vi "Do.vi"(8 "error in (no error)":errorcluster, 10 "Actor in":refnum<class "Actor.lvclass">, 11 "Initialize Msg":refnum<class "Initialize Work Msg.lvclass">) -> (0 "error out":errorcluster, 2 "Actor out":refnum<class "Actor.lvclass">)   [LabVIEW 2021, in "Initialize Work Msg.lvclass"]
doc: "This VI delivers the message to the actor by calling the appropriate method(s) on the actor."
uses:
  Initialize Work Msg.lvclass
  Initialize Work Msg.lvclass/Initialize Work Msg.ctl
  Woker Interface/Worker.lvclass
  38615d65-fe0a-408a-ba5f-f88dbd155317.vi
  <vilib>/ActorFramework/Actor/Actor.lvclass
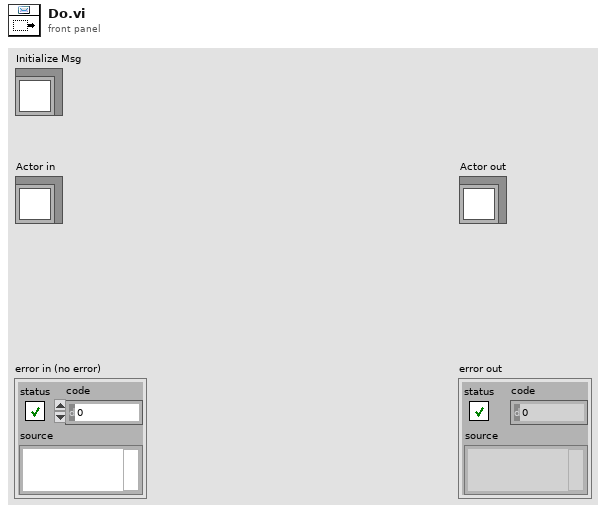
[diagram p1: front panel]
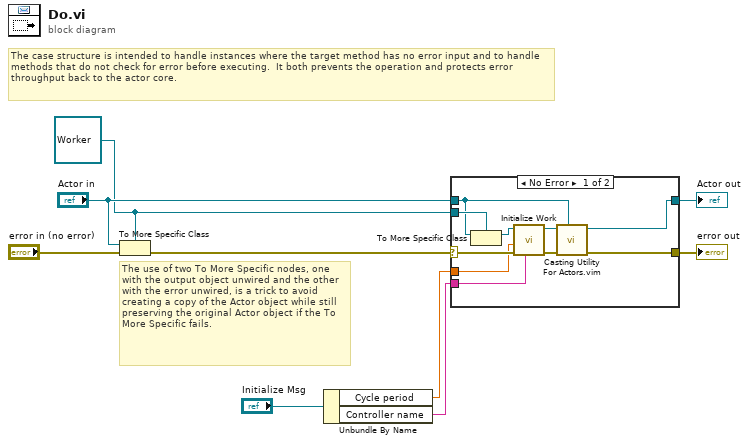
[diagram p0: block diagram]
diagram:
  w4 = refnum<class "Worker.lvclass"> refnum ("Actor in")
  # "The use of two To More Specific nodes, one with the output object unwired and the other with the error unwired, is a trick to avoid creating a copy of the Actor object while still preserving the original Actor object if the To More Specific fails."
  # "The case structure is intended to handle instances where the target method has no error input and to handle methods that do not check for error before executing.  It both prevents the operation and protects error throughput back to the actor core."
  n1 = To More Specific Class(target class=w4, reference="Actor in", error in="error in (no error)") -> (error out=w8:errorcluster)  [unwired: 1 out]
  n2 = Unbundle By Name("Initialize Msg") -> ("Cycle period"=w2:dbl, "Controller name"=w1:string)
  n3 = case shown="No Error" w8 {
    selector: w8 -> [w19 w21]
    tunnel: [w13 w21] -> w7
    tunnel: [w11 w20] -> w6
    tunnel: "Actor in" -> [w10 w20]
    tunnel: w4 -> [w18 _]
    tunnel: w2 -> [w16 _]
    tunnel: w1 -> [w15 _]
    frame No Error {
      n4 = To More Specific Class(target class=w18, reference=w10) -> (specific class reference=w17:refnum<class "Worker.lvclass">)  [unwired: 1 in, 1 out]
      n5 = call-dynamic "Initialize Work.vi"("Controller name"=w15, "error in (no error)"=w19, "Update period"=w16, "Worker in"=w17) -> ("error out"=w14:errorcluster, "Worker out"=w12:refnum<class "Worker.lvclass">)  [unwired: 6 in]
      n6 = call "Casting Utility For Actors.vim"("type"=w10, "error in (no error)"=w14, "Actor in"=w12) -> ("error out"=w13:errorcluster, "Actor out"=w11:refnum<class "Actor.lvclass">)  [unwired: 7 in]
    }
    frame Error {
      # "If type check fails, pass the original object out again."
    }
  }
  "error out" <- w7
  "Actor out" <- w6
